vi "Generate Event.vi"(4 "Error In":errorcluster, 5 "Response Notifier":string, 6 "TC Parameters":T1, 7 "Plugin Name":string) -> (0 "Error Out":errorcluster)   [LabVIEW 2015, in "Set TC Parameters.lvlib"]
uses:
  Set TC Parameters.lvlib
  _libraries/Startup Processes/_typedefs/TC Setup Parameters.ctl
  _typedefs/Event Data.ctl
  _libraries/Startup Processes/Startup Processes.lvlib
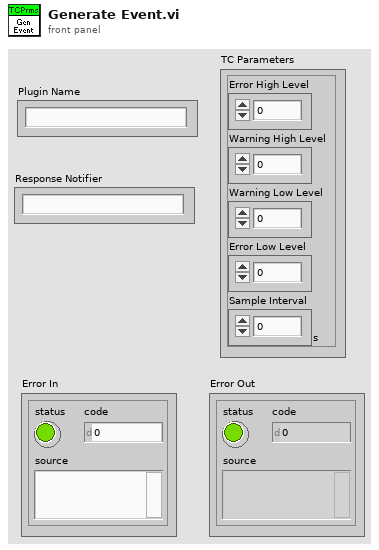
[diagram p1: front panel]
types:
  T1 = typedef "Startup Processes.lvlib/TC Setup Parameters.ctl" = cluster{"Error High Level":dbl, "Warning High Level":dbl, "Warning Low Level":dbl, "Error Low Level":dbl, "Sample Interval":dbl[unit]}
  T2 = typedef "Set TC Parameters.lvlib/Event Data.ctl" = cluster{"Plugin Name":string, "TC Parameters":T1, "Response Notifier":string}
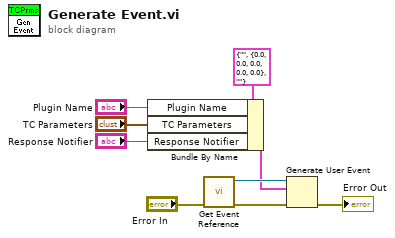
[diagram p0: block diagram]
diagram:
  n1 = Bundle By Name(cluster=T2 {"Plugin Name"="", "TC Parameters"={"Error High Level"=0.0, "Warning High Level"=0.0, "Warning Low Level"=0.0, "Error Low Level"=0.0, "Sample Interval"=0.0}, "Response Notifier"=""} ("event data"), "Plugin Name"="Plugin Name", "TC Parameters"="TC Parameters", "Response Notifier"="Response Notifier") -> (w4:T2)
  n2 = call "Get Event Reference.vi"("error in (no error)"="Error In") -> ("error out"=w8:errorcluster, "Set TC Parameters"=w7:refnum<user-event>)  [unwired: 5 in]
  n3 = Generate User Event(user event=w7, event data cluster=w4, error in=w8) -> (error out=→"Error Out":errorcluster)  [unwired: 1 in, 1 out]
